vi "setFrequency.vi"(7 "Channel":string="0", 8 "error in (no error)":errorcluster, 10 "Frequency [Hz]":dbl, 11 "Fgen in":refnum<class "Arb.lvclass">) -> (0 "error out":errorcluster, 3 "Fgen out":refnum<class "Arb.lvclass">)   [LabVIEW 2023, in "sweArb.lvlib" / "Arb.lvclass"]
doc: "<b>Author:</b> Wolfgang\n<b>Description:</b> Set Output Frequency in Hz"
uses:
  Arb.lvclass
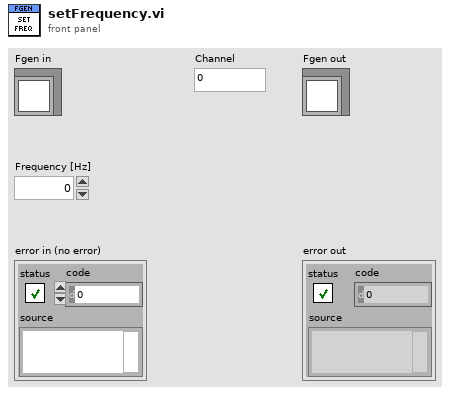
[diagram p1: front panel]
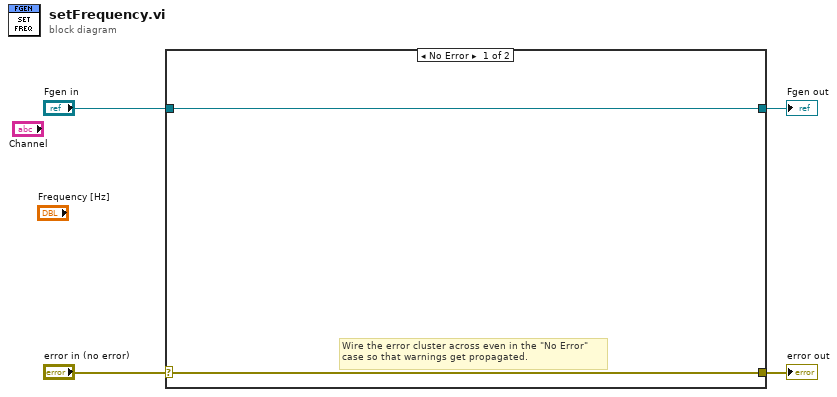
[diagram p0: block diagram]
diagram:
  n1 = case shown="No Error" "error in (no error)" {
    selector: "error in (no error)" -> [w5 w8]
    tunnel: [w5 w8] -> w3
    tunnel: [w6 w7] -> w1
    tunnel: "Fgen in" -> [w6 w7]
    frame No Error {
      # "Wire the error cluster across even in the \"No Error\"\ncase so that warnings get propagated."
    }
    frame Error {
    }
  }
  "error out" <- w3
  "Fgen out" <- w1
